vi "Update Current Temperature.vi"(8 "error in (no error)":errorcluster, 10 "Current Temperature":dbl, 11 "Cooler Controller in":refnum<class "Cooler Controller.lvclass">) -> (0 "error out":errorcluster, 3 "Cooler Controller out":refnum<class "Cooler Controller.lvclass">)   [LabVIEW 2025, in "Cooler Controller.lvlib" / "Cooler Controller.lvclass"]
doc: "Child classes must override this method to read a sensor or simulated source for the current temperature of the system."
uses:
  Cooler Controller.lvclass
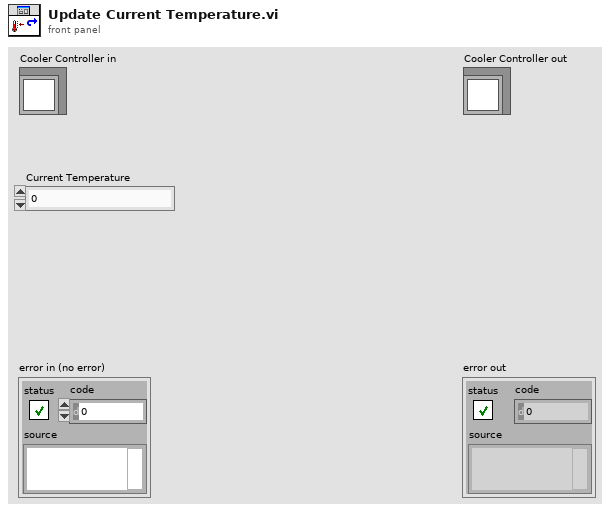
[diagram p1: front panel]
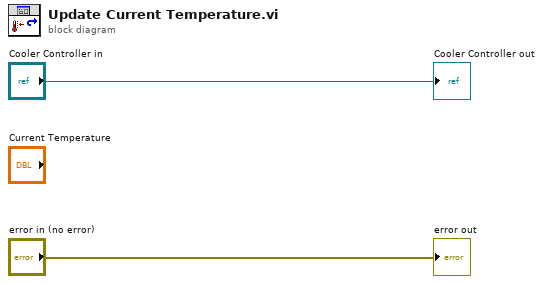
[diagram p0: block diagram]
diagram:
  "error out" <- "error in (no error)"
  "Cooler Controller out" <- "Cooler Controller in"
